vi "CreatePublicEvents.vi"(8 "error in (no error)":errorcluster, 11 "Analyzer":refnum<class "Analyzer.lvclass">) -> (0 "error out":errorcluster, 3 "Analyzer out":refnum<class "Analyzer.lvclass">)   [LabVIEW 2022 SP3, in "Analyzer.lvclass"]
uses:
  Analyzer.lvclass
  Analyzer.lvclass/Analyzer.ctl
  Typedefs/Analyzer State--enum.ctl
  Typedefs/PublicEvents--Cluster.ctl
  Typedefs/PublicEvents--Analyzer.NewEventMessage.ctl
  <vilib>/JKI/JKI SMO/SMO/SMO.lvclass
panel:
  # "For instructions on how to use the JKI State Machine Objects, examples and video tutorials, visit:\nhttp://jki.net/state-machine-objects/\n\nJKI State Machine Objects™\nhttp://jki.net/state-machine-objects/\nCopyright (C) 2005-2015, JKI <info@jki.net>\nALL RIGHTS RESERVED"
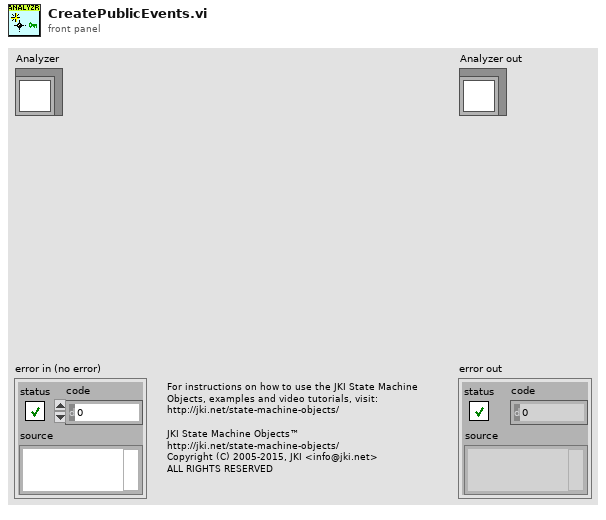
[diagram p1: front panel]
types:
  T1 = typedef "Analyzer.lvclass/PublicEvents--Cluster.ctl" = cluster{"UI State":refnum<user-event>, "NewEventMessage":refnum<user-event>}
  T2 = typedef "Analyzer.lvclass/Analyzer State--enum.ctl" = enum16{"unknown", "Opened", "Embedded", "Closed"}
  T3 = typedef "Analyzer.lvclass/PublicEvents--Analyzer.NewEventMessage.ctl" = cluster{"Title":string}
  T4 = typedef "Analyzer.lvclass/PrivateData--Ref.ctl" = refnum<data-value>
  T5 = typedef "Analyzer.lvclass/PrivateData--Cluster.ctl" = cluster{"Public Events":T1, "Subpanel Ref":refnum<vi>, "UI State":T2}
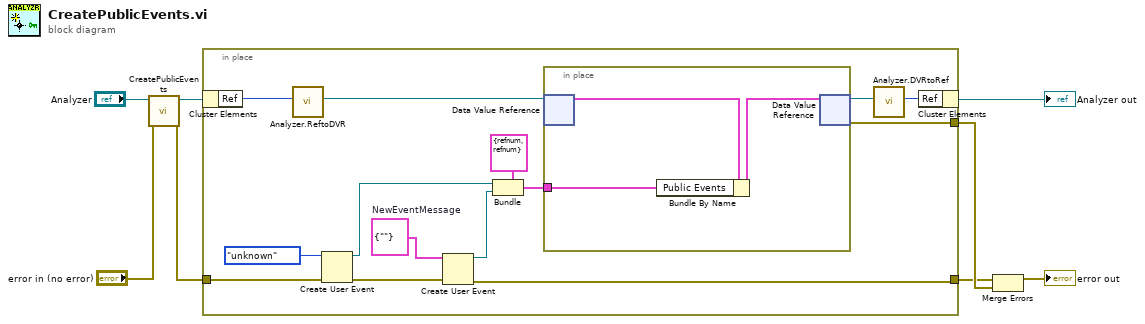
[diagram p0: block diagram]
diagram:
  n1 = call-parent "CreatePublicEvents.vi"("error in (no error)"="error in (no error)", "SMO"="Analyzer") -> ("error out"=w2:errorcluster, "SMO out"=w3:refnum<class "Analyzer.lvclass">)  [unwired: 8 in]
  n2 = in-place {
    in-place-border: [w22] -> w8
    in-place-border: w2 -> [w14]
    in-place-border: [w11] -> w1
    w9 = T3 {"Title"=""}  # NewEventMessage
    n3 = in-place-cluster #1(w3) -> ("Ref"=w21:u32)
    n4 = call "Analyzer.ReftoDVR.vi"("Ref"=w21) -> ("Ref"=w20:T4)  [unwired: 10 in]
    n5 = Create User Event(user event datatype=Analyzer_State--enum."unknown" ("UI State"), error in=w14) -> (user event=w16:refnum<user-event>, error out=w12:errorcluster)
    n6 = Create User Event(user event datatype=w9, error in=w12) -> (user event=w10:refnum<user-event>, error out=w11:errorcluster)
    n7 = Bundle(cluster=T1 {"UI State"=refnum, "NewEventMessage"=refnum} ("Public Events"), "UI State"=w16, "NewEventMessage"=w10) -> (w19:T1)
    n8 = in-place {
      in-place-border: w19 -> [w23]
      n9 = in-place-dvr #2(w20) -> (w25:T5)  [unwired: 1 out]
      n10 = Bundle By Name(cluster=w25, "Public Events"=w23) -> (w24:T5)
      n11 = in-place-dvr #2(w24) -> (w18:T4, w22:errorcluster)
    }
    n12 = call "Analyzer.DVRtoRef.vi"("Ref"=w18) -> ("Ref"=w17:u32)  [unwired: 10 in]
    n13 = in-place-cluster #1("Ref"=w17) -> (→"Analyzer out":refnum<class "Analyzer.lvclass">)
  }
  n14 = Merge Errors(w1, w8) -> (→"error out":errorcluster)
